vi "IsLanguagePresent.vi"(8 "error in":errorcluster, 10 "Target Language":string, 11 "Languages":T1[](array[typedef])) -> (0 "error out":errorcluster, 2 "Target Language Present?":bool)   [LabVIEW 2017, in "JKI Simple Localization.lvlib"]
uses:
  API/JKI Simple Localization.lvlib
  Definitions/Private/Font -- Cluster.ctl
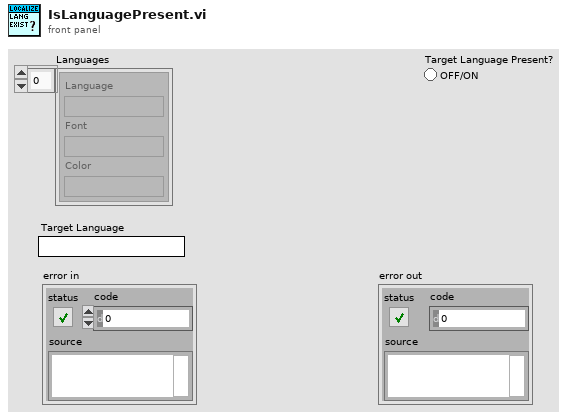
[diagram p1: front panel]
types:
  T1 = typedef "JKI Simple Localization.lvlib/Font -- Cluster.ctl" = cluster{"Language":string, "Font":string, "Color":string}
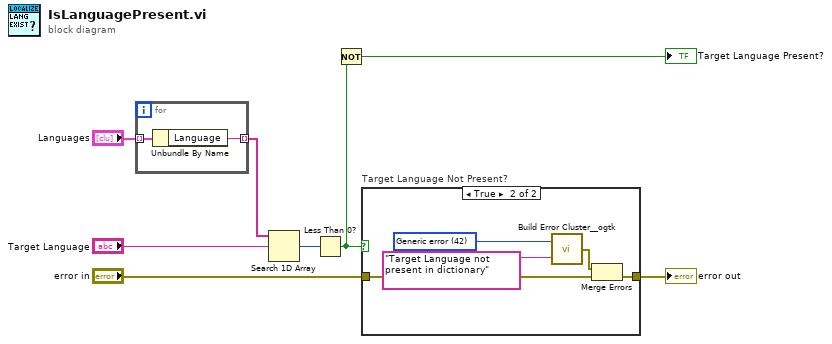
[diagram p0: block diagram]
diagram:
  n1 = for {
    tunnel: "Languages" -> [w10] mode=indexing
    tunnel: [w9] -> w1 mode=indexing
    n2 = Unbundle By Name(w10) -> ("Language"=w9:string)
  }
  n3 = Search 1D Array(1D array=w1, element="Target Language") -> (index of element=w7:i32)  [unwired: 1 in]
  n4 = Less Than 0?(x=w7) -> (x < 0?=w4:bool)
  n5 = Not(x=w4) -> (.not. x?=→"Target Language Present?":bool)
  n6 = case "Target Language Not Present?" shown="True" w4 {
    tunnel: "error in" -> [w11 w13]
    tunnel: [w11 w12] -> w6
    frame False {
    }
    frame True {
      w16 = 42 items=["No error", "Argument error", "Memory is full", "Out of zone", "End of file", "File already open", "Generic file I/O error", "File not found", "File permission error", "Disk is full", "Duplicate path", "Too many files open", "System feature not enabled", "Resource file not found", "Cannot add resource", "Resource not found", "Image not found", "Image memory error", "Pen does not exist", "Config type invalid", "Config token not found", "Config parse error", "Config memory error", "Bad external code format", "Bad external code offset", "External code not present", "Null window", "Destroy window error", "Null menu", "Print aborted", "Bad print record", "Print driver error", "Windows error during printing", "Memory error during printing", "Print dialog error", "Generic print error", "Invalid device refnum", "Device not found", "Device parameter error", "Device unit error", "Cannot open device", "Device call aborted", "Generic error", "Cancelled by user", "Object ID too low", "Object ID too high", "Object not in heap", "Unknown heap", "Unknown object (invalid DefProc)", "Unknown object (DefProc not in table)", "Message out of range", "Invalid (null) method", "Unknown message", "Manager call not supported", "Bad address", "Network operation in progress", "Network operation timed out", "Connection is busy", "Network attribute not supported", "Network error", "Address in use", "System out of memory", "Connection aborted", "Connection refused", "Not connected", "Already connected", "Connection closed", "Initialization error (interapplication manager)", "Bad occurrence", "Wait on unbound occurrence handler", "Occurrence queue overflow", "Datalog type conflict", "Unused", "Unrecognized type (interapplication manager)", "Memory corrupt", "Failed to make temporary DLL", "Old CIN version", "Drag socket not found", "Failed to load drop-object", "Failed to register OLE object", "Failed to release OLE object", "Format specifier type mismatch", "Unknown format specifier", "Too few format specifiers", "Too many format specifiers", "Scan failed", "Newer CIN version", "Error converting to variant", "Runtime menu error", "Password tampered", "Variant attribute not found", "Incompatible variant data type", "Event data is not available", "Event Store is not present", "Occurrence is not found", "Event Queue is not created", "Event info is not available", "Refnum passed is NULL", "Error retrieving Class GUID", "Error retrieving CoClass GUID", "Error retrieving TypeLib GUID.", "Bad built application magic bytes.", "Specific driver is different from the specific driver associated with the Logical Name.", "There is no session opened to the class driver.", "Max Error", "MAX - Error with config objects", "MAX - Error loading configuration", "MAX - Group not supported"]
      n7 = call <userlib>:"Build Error Cluster__ogtk.vi"("String to Prepend to source (\"\")"="Target Language not present in dictionary" ("String to Prepend to source (\"\")"), "code"=w16) -> ("error out"=w14:errorcluster)
      n8 = Merge Errors(w14, w13) -> (w12:errorcluster)
    }
  }
  "error out" <- w6
